vi "Close Log.vi"(8 "error in (no error)":errorcluster, 11 "Model in":refnum<class "Model.lvclass">) -> (0 "error out":errorcluster, 3 "Model out":refnum<class "Model.lvclass">)   [LabVIEW 2016, in "Model.lvclass"]
uses:
  Model.lvclass
  Model.lvclass/Model.ctl
  Test Log/Test Log/OperationsLog.lvclass
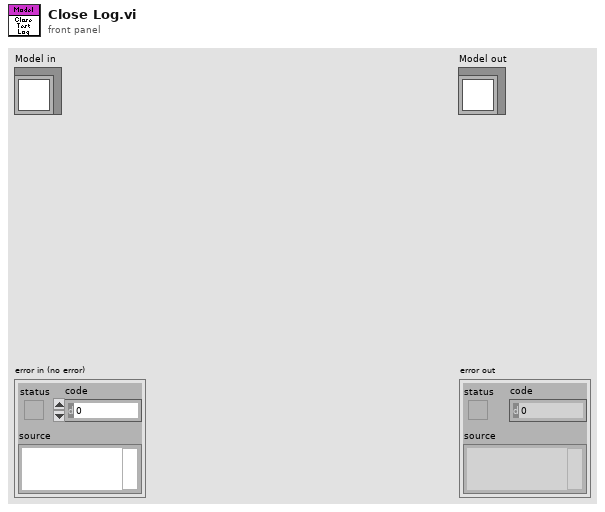
[diagram p1: front panel]
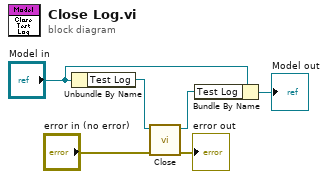
[diagram p0: block diagram]
diagram:
  n1 = Unbundle By Name("Model in") -> ("Test Log"=w4:refnum<class "OperationsLog.lvclass">)
  n2 = call-dynamic "Close.vi"("error in (no error)"="error in (no error)", "Test Log in"=w4) -> ("error out"=→"error out":errorcluster, "Test Log out"=w1:refnum<class "OperationsLog.lvclass">)  [unwired: 8 in]
  n3 = Bundle By Name(cluster="Model in", "Test Log"=w1) -> (→"Model out":refnum<class "Model.lvclass">)
